vi "4155C Output.vi"(0 "VISA resource name in":refnum<visa-resource-name>="GPIB0::14::INSTR", 2 "Gate":T5={"Gate Start"=0.0, "Gate Stop"=0.0, "Gate Step"=0.0, "Gate Compliance"=0.1, "Gate PComp"=0.0, "Range mode"=0, "Range"=6} {"Range" max=11 scale=0.0..11.0; "Range mode" items=["Auto", "Limited", "Fixed"]; "Gate PComp" format="%^.2e"; "Gate Compliance" format="%^.2e"; "Gate Step" format="%^.4e"; "Gate Stop" format="%^.4e"; "Gate Start" format="%^.4e"}, 3 "Drain":T6={"Drain Start"=0.0, "Drain Stop"=0.0, "Drain Compliance"=0.1, "Drain Step (linear only)"=0.0, "Drain PComp"=0.0, "Range mode"=0, "Range"=6} {"Range" max=11 scale=0.0..11.0; "Range mode" items=["Auto", "Limited", "Fixed"]; "Drain PComp" format="%^.2e"; "Drain Step (linear only)" format="%^.4e"; "Drain Compliance" format="%^.2e"; "Drain Stop" format="%^.4e"; "Drain Start" format="%^.4e"}, 5 "Timings":T4={"integration time"=0, "Short/Long integration time"=0.00064, "hold time (sec)"=0.0, "delay time (sec)"=0.0, "Step Time (0 disables)"=0.0, "sweep method"=0, "Pulse period"=0.005, "Base voltage"=0.0, "Pulse width"=0.0005} {"Pulse width" min=0.0005 max=0.1 step=0.0001 format="%.4f"; "Base voltage" format="%^.4e"; "Pulse period" min=0.005 max=1.0 step=0.0001 format="%.4f"; "sweep method" items=["Continuous", "Pulsed"]; "Step Time (0 disables)" format="%.2f"; "delay time (sec)" format="%.4f"; "hold time (sec)" format="%.4f"; "Short/Long integration time" format="%^.0e"; "integration time" scale=0.0..2.0}, 6 "error in (no error)":errorcluster, 7 "SMU4":cluster{"on/off":bool, "Voltage":dbl} {"Voltage" min=-100.0 max=100.0 format="%.2f"}, 10 "sweep mode":u16(ring) items=["Single", "Double"], 12 "Panel controls":T3={"Emergency Stop"=refnum, "OutputGraph Max"=1e-05, "Text/Graph (text=false)"=FALSE} {"OutputGraph Max" format="%.2e"}, 13 "Standby":T1) -> (16 "VD":dbl[](array[numeric]) format="%.2f", 17 "Outparams":T2={"V2 Start"=0.0, "V2 Step"=0.0, "Number of points"=1} {"V2 Step" format="%.2f"; "V2 Start" format="%^.4e"}, 20 "VISA Resource Name out":refnum<visa-resource-name>, 22 "IS":dbl[](array[numeric]) format="%.2f", 23 "ID":dbl[](array[numeric]) format="%.2f", 25 "IG":dbl[](array[numeric]) format="%.2f", 26 "error out":errorcluster, 27 "SMU4":dbl[](array[numeric]) format="%.2f")   [LabVIEW 2016]
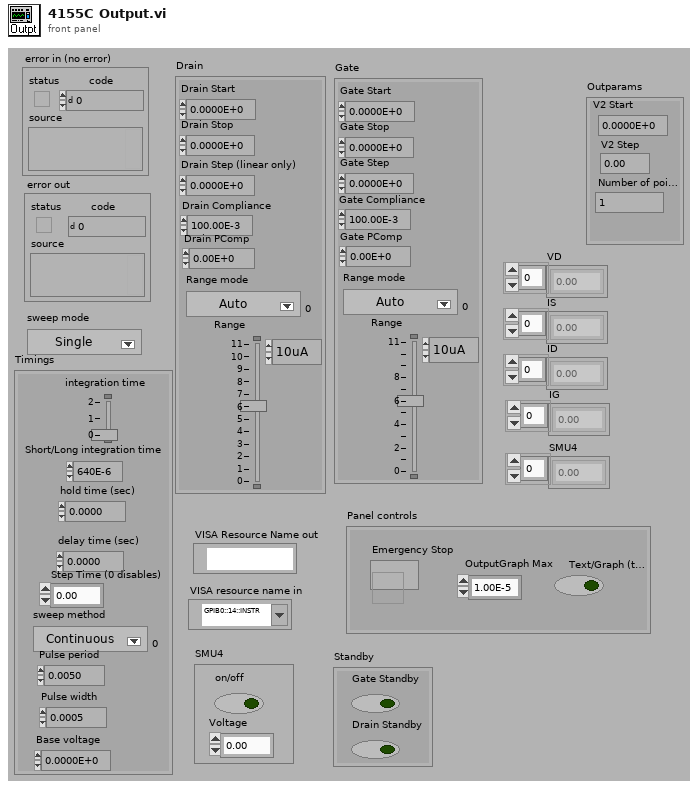
[diagram p1: front panel]
types:
  T1 = cluster{"Gate Standby":bool, "Drain Standby":bool}
  T2 = cluster{"V2 Start":dbl, "V2 Step":dbl, "Number of points":i32}
  T3 = cluster{"Emergency Stop":refnum<vi>, "OutputGraph Max":dbl, "Text/Graph (text=false)":bool}
  T4 = cluster{"integration time":u32, "Short/Long integration time":dbl, "hold time (sec)":dbl, "delay time (sec)":dbl, "Step Time (0 disables)":dbl, "sweep method":u16, "Pulse period":dbl, "Base voltage":dbl, "Pulse width":dbl}
  T5 = cluster{"Gate Start":dbl, "Gate Stop":dbl, "Gate Step":dbl, "Gate Compliance":dbl, "Gate PComp":dbl, "Range mode":u16, "Range":u8}
  T6 = cluster{"Drain Start":dbl, "Drain Stop":dbl, "Drain Compliance":dbl, "Drain Step (linear only)":dbl, "Drain PComp":dbl, "Range mode":u16, "Range":u8}
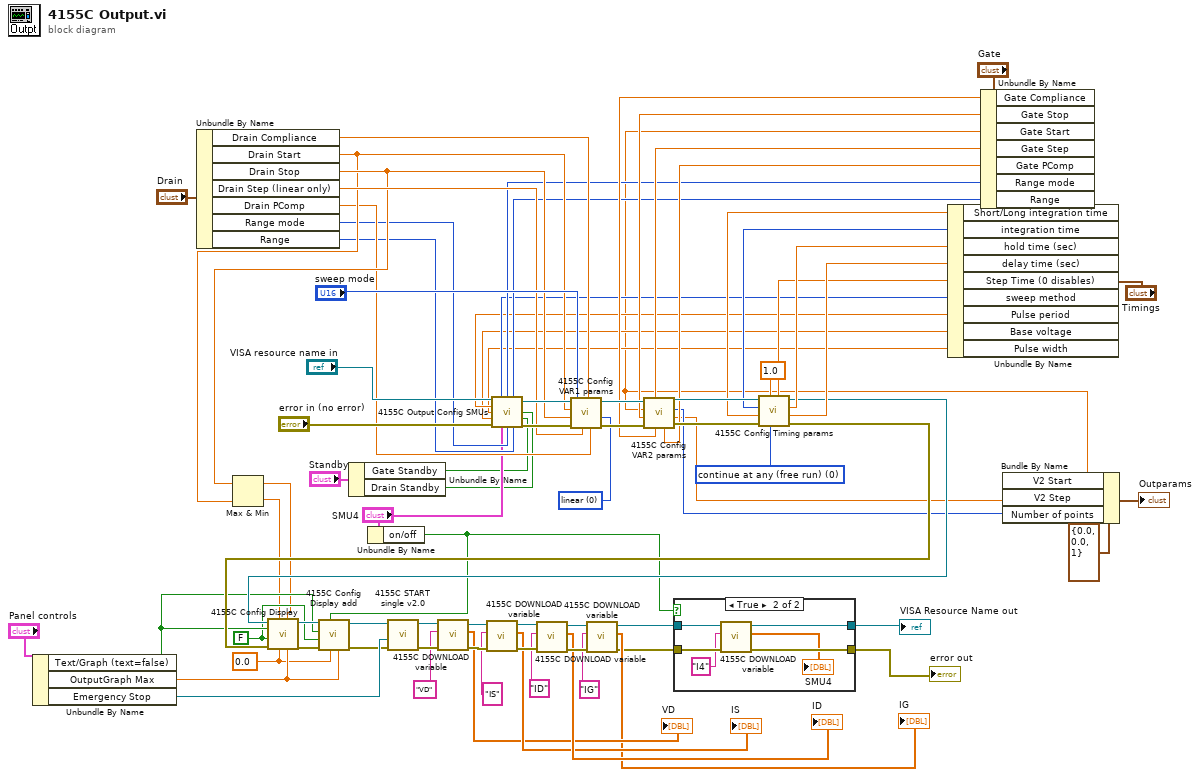
[diagram p0: block diagram]
diagram:
  w4 = 0.0 ("Ymin")
  w5 = FALSE ("Logarithmic")
  w65 = u8 0 items=["continue at any (free run)", "stop at any abnorm", "stop at compliance"] ("stop condition (free run:0)")
  w62 = u16 0 items=["linear", "log 10", "log 25", "log 50"] ("sweep spacing (linear: 0)")
  n1 = Unbundle By Name("Panel controls") -> ("Text/Graph (text=false)"=w6:bool, "OutputGraph Max"=w7:dbl, "Emergency Stop"=w35:refnum<vi>)
  n2 = Unbundle By Name("Drain") -> ("Drain Compliance"=w49:dbl, "Drain Start"=w37:dbl, "Drain Stop"=w38:dbl, "Drain Step (linear only)"=w48:dbl, "Drain PComp"=w34:dbl, "Range mode"=w30:u16, "Range"=w29:u8)
  n3 = Max & Min(x=w38, y=w37) -> (max(x,y)=w2:dbl, min(x,y)=w3:dbl)
  n4 = Unbundle By Name("Standby") -> ("Gate Standby"=w12:bool, "Drain Standby"=w13:bool)
  n5 = Unbundle By Name("SMU4") -> ("on/off"=w1:bool)
  n6 = Unbundle By Name("Timings") -> ("Short/Long integration time"=w67:dbl, "integration time"=w44:u32, "hold time (sec)"=w45:dbl, "delay time (sec)"=w46:dbl, "Step Time (0 disables)"=w41:dbl, "sweep method"=w28:u16, "Pulse period"=w27:dbl, "Base voltage"=w25:dbl, "Pulse width"=w26:dbl)
  n7 = Unbundle By Name("Gate") -> ("Gate Compliance"=w52:dbl, "Gate Stop"=w51:dbl, "Gate Start"=w20:dbl, "Gate Step"=w50:dbl, "Gate PComp"=w33:dbl, "Range mode"=w32:u16, "Range"=w31:u8)
  n8 = call "4155C Output Config SMUs.vi"("VISA resource name in"="VISA resource name in", "sweep method"=w28, "Gate mode"=w32, "Gate Range"=w31, "Pulse period"=w27, "Pulse width"=w26, "Drain Standby"=w13, "Base voltage"=w25, "Gate Standby"=w12, "error in (no error)"="error in (no error)", "SMU4"="SMU4", "Source/drain mode"=w30, "Source/drain Range"=w29) -> ("VISA Resource Name out"=w60:refnum<visa-resource-name>, "error out"=w59:errorcluster)  [unwired: 1 in]
  n9 = call "4155C Config VAR1 params.vi"("sweep spacing (linear: 0)"=w62, "power compliance (0 = OFF)"=w34, "compliance"=w49, "step (linear only)"=w48, "sweep mode"="sweep mode", "error in (no error)"=w59, "stop"=w38, "start"=w37, "VISA session"=w60) -> ("error out"=w63:errorcluster, "dup VISA resource name"=w64:refnum<visa-resource-name>)  [unwired: 1 out]
  n10 = call "4155C Config VAR2 params.vi"("power compliance (0 = OFF)"=w33, "compliance"=w52, "step"=w50, "error in (no error)"=w63, "stop"=w51, "start"=w20, "VISA session"=w64) -> ("error out"=w68:errorcluster, "Corrected Step"=w21:dbl, "Number of points"=w22:i32, "dup VISA resource name"=w69:refnum<visa-resource-name>)  [unwired: 1 in]
  n11 = call "4155C Config Timing params.vi"("delay time (sec)"=w46, "hold time (sec)"=w45, "Step Time (0 disables)"=w41, "stop condition (free run:0)"=w65, "wait time parameter"=1.0, "error in (no error)"=w68, "Short/Long integration time"=w67, "integration time"=w44, "VISA session"=w69) -> ("error out"=w40:errorcluster, "dup VISA resource name"=w39:refnum<visa-resource-name>)  [unwired: 1 in]
  n12 = call "4155C Config Display.vi"("Ymax"=w7, "Var1 Stop"=w2, "Ymin"=w4, "Var1 Start"=w3, "error in (no error)"=w40, "Logarithmic"=w5, "SPA Display"=w6, "VISA session"=w39) -> ("error out"=w8:errorcluster, "dup VISA resource name"=w11:refnum<visa-resource-name>)  [unwired: 2 in]
  n13 = call "4155C Config Display add.vi"("Ymax"=w7, "Ymin"=w4, "SMU4"=w1, "error in (no error)"=w8, "Logarithmic"=w5, "SPA Display"=w6, "VISA session"=w11) -> ("error out"=w9:errorcluster, "dup VISA resource name"=w10:refnum<visa-resource-name>)  [unwired: 3 in]
  n14 = call "4155C START single v2.0.vi"("error in (no error)"=w9, "Emergency Stop"=w35, "VISA resource name in"=w10) -> ("error out"=w80:errorcluster, "VISA Resource Name out"=w81:refnum<visa-resource-name>)  [unwired: 3 in]
  n15 = call "4155C DOWNLOAD variable.vi"("error in (no error)"=w80, "Variable name"="VD", "VISA resource name in"=w81) -> ("error out"=w78:errorcluster, "Output data"=→"VD":dbl[], "VISA Resource Name out"=w77:refnum<visa-resource-name>)  [unwired: 2 in]
  n16 = call "4155C DOWNLOAD variable.vi"("error in (no error)"=w78, "Variable name"="IS", "VISA resource name in"=w77) -> ("error out"=w74:errorcluster, "Output data"=→"IS":dbl[], "VISA Resource Name out"=w75:refnum<visa-resource-name>)  [unwired: 2 in]
  n17 = call "4155C DOWNLOAD variable.vi"("error in (no error)"=w74, "Variable name"="ID", "VISA resource name in"=w75) -> ("error out"=w73:errorcluster, "Output data"=→"ID":dbl[], "VISA Resource Name out"=w72:refnum<visa-resource-name>)  [unwired: 2 in]
  n18 = call "4155C DOWNLOAD variable.vi"("error in (no error)"=w73, "Variable name"="IG", "VISA resource name in"=w72) -> ("error out"=w15:errorcluster, "Output data"=→"IG":dbl[], "VISA Resource Name out"=w18:refnum<visa-resource-name>)  [unwired: 2 in]
  n19 = case shown="True" w1 {
    tunnel: w18 -> [w83 w89]
    tunnel: [w83 w86] -> w17
    tunnel: [w82 w87] -> w16
    tunnel: w15 -> [w82 w88]
    frame False {
    }
    frame True {
      n20 = call "4155C DOWNLOAD variable.vi"("error in (no error)"=w88, "Variable name"="I4", "VISA resource name in"=w89) -> ("error out"=w87:errorcluster, "Output data"=→"SMU4":dbl[], "VISA Resource Name out"=w86:refnum<visa-resource-name>)  [unwired: 2 in]
    }
  }
  "error out" <- w16
  "VISA Resource Name out" <- w17
  n21 = Bundle By Name(cluster=T2 {"V2 Start"=0.0, "V2 Step"=0.0, "Number of points"=1} ("Outparams"), "V2 Start"=w20, "V2 Step"=w21, "Number of points"=w22) -> (→"Outparams":T2)
